vi "Page_Destination_Update_Display.vi"(8 "error in (no error)":errorcluster, 9 "ctlReferences":T1, 11 "AB_Destination in":refnum<class "AB_Destination.lvclass">) -> (0 "error out":errorcluster, 3 "AB_Destination out":refnum<class "AB_Destination.lvclass">)   [LabVIEW 2020, in "AB_Destination.lvclass"]
uses:
  <vilib>/AppBuilder/AB_Classes/Destination/AB_Destination.lvclass
  <resource>/Framework/Providers/Builds/AppBuilder/AB_UI_Page_Destination_References.ctl
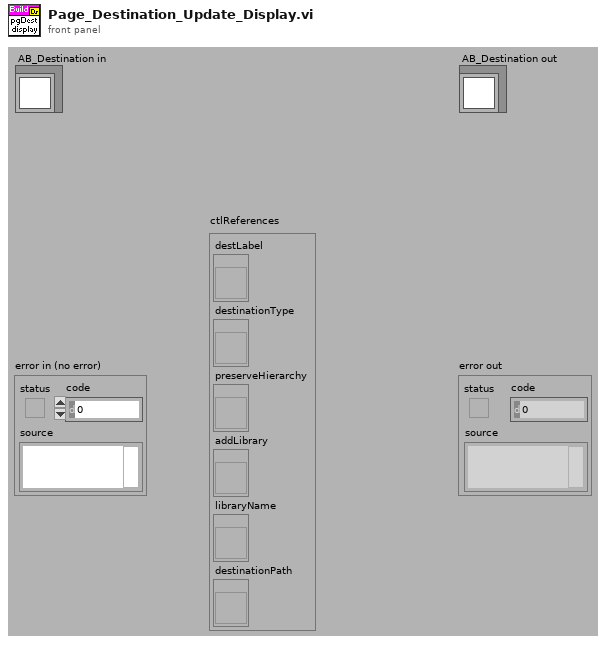
[diagram p1: front panel]
types:
  T1 = typedef "AB_UI_Page_Destination_References.ctl" = cluster{"destLabel":refnum<vi>, "destinationType":refnum<vi>, "preserveHierarchy":refnum<vi>, "addLibrary":refnum<vi>, "libraryName":refnum<vi>, "destinationPath":refnum<vi>}
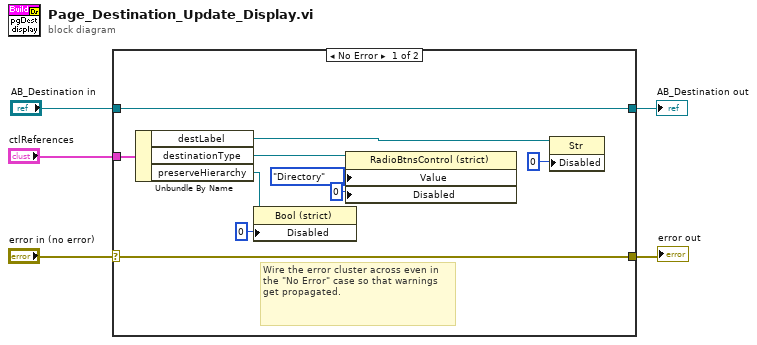
[diagram p0: block diagram]
diagram:
  n1 = case shown="No Error" "error in (no error)" {
    selector: "error in (no error)" -> [w14 w17]
    tunnel: [w14 w17] -> w4
    tunnel: [w15 w16] -> w2
    tunnel: "AB_Destination in" -> [w15 w16]
    tunnel: "ctlReferences" -> [w12 _]
    frame No Error {
      # "Wire the error cluster across even in the \"No Error\" case so that warnings get propagated."
      n2 = Unbundle By Name(w12) -> ("destLabel"=w9:refnum<vi>, "destinationType"=w11:refnum<vi>, "preserveHierarchy"=w7:refnum<vi>)
      n3 = property class="Bool (strict)"(reference=w7, "Disabled"=u8 0) -> ()  [unwired: 1 in, 2 out]
      n4 = property class="RadioBtnsControl (strict)"(reference=w11, "Value"=enum32{"No Selection", "Directory", "LLB"}."Directory", "Disabled"=u8 0) -> ()  [unwired: 1 in, 2 out]
      n5 = property class="Str"(reference=w9, "Disabled"=u8 0) -> ()  [unwired: 1 in, 2 out]
    }
    frame Error {
    }
  }
  "error out" <- w4
  "AB_Destination out" <- w2
